vi "niFPGA BW CU Order 1.vi"   [LabVIEW 2017]
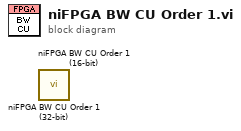
[diagram p0: block diagram]
diagram:
  n1 = call <vilib>:"niFPGA BW CU Order 1 (32-bit).vi"() -> ()  [unwired: 11 in, 5 out]
  n2 = call <vilib>:"niFPGA BW CU Order 1 (16-bit).vi"() -> ()  [unwired: 11 in, 5 out]
